vi "Test_NetworkStream Handshake.vi"() -> ()   [LabVIEW 2013]
uses:
  <vilib>/LabVIEW Open Source Project/OpenURI/utilities/Extract URI Components.vi
  <vilib>/Utility/error.llb/Trim Whitespace.vi
  <vilib>/LabVIEW Open Source Project/Unicity/RandomStringGenerator/RandomStringGenerator.lvclass
  <vilib>/LabVIEW Open Source Project/OpenURI/openURI.lvlib
panel:
  out "State verfied":bool
  out "Echo":string
  out "Echo verfied":bool
  out "Auth Ack/Nack":string
  out "Challenge verified":bool
  out "error out 2":errorcluster
  out "error out":errorcluster
  out "Client Reader":string
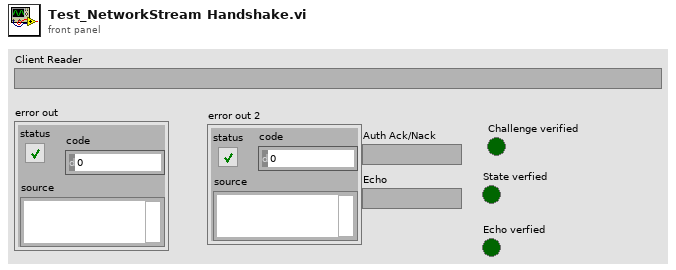
[diagram p1: front panel]
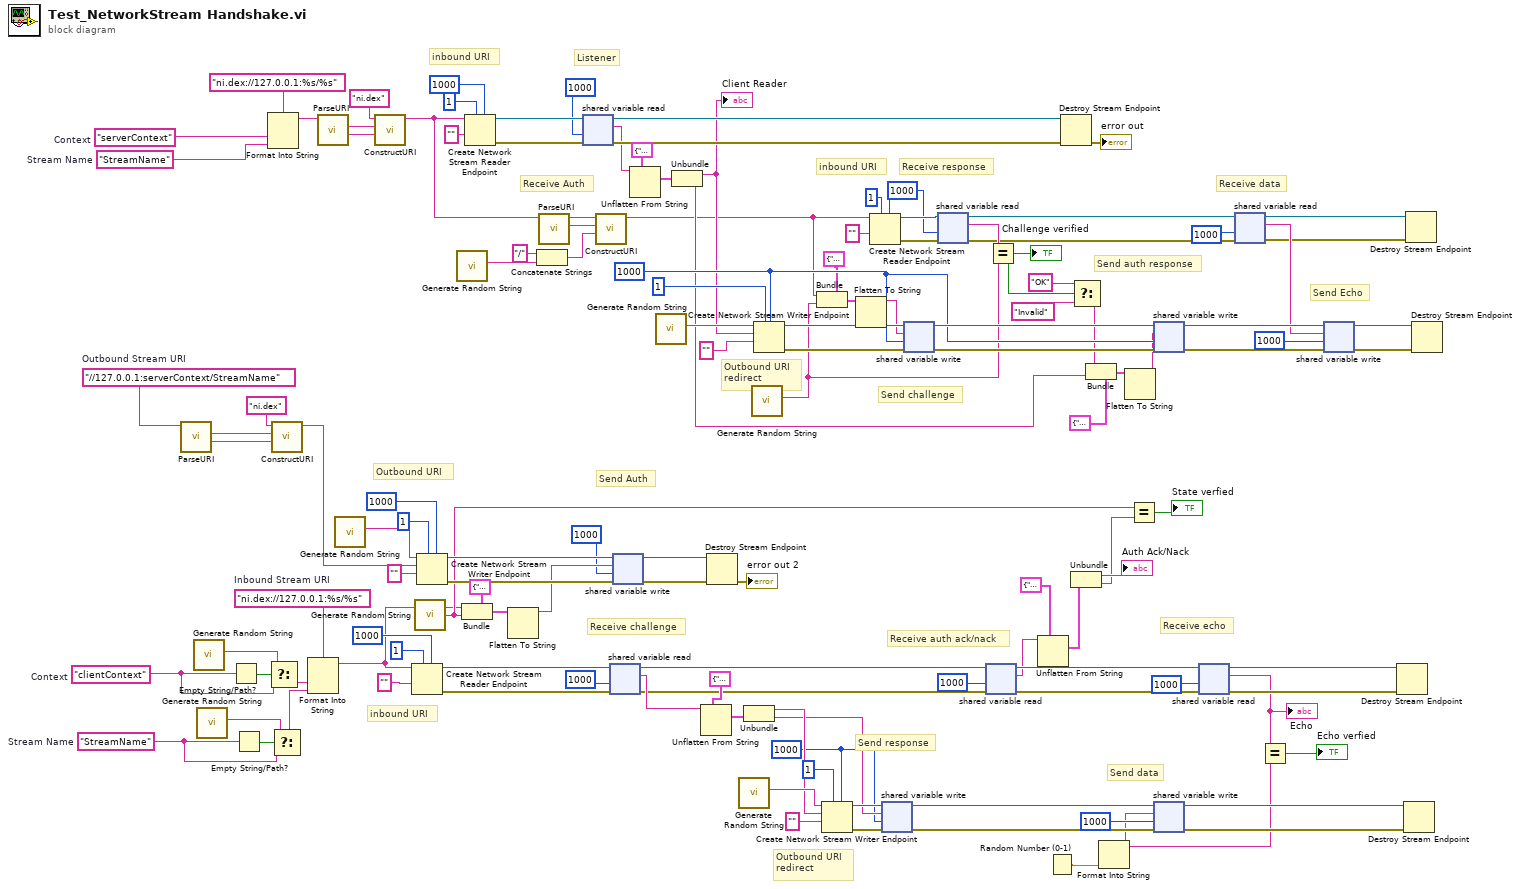
[diagram p0: block diagram]
diagram:
  w18 = "ni.dex://127.0.0.1:%s/%s"  # Inbound Stream URI
  w14 = "StreamName"  # Stream Name
  w9 = "clientContext"  # Context
  w20 = "StreamName"  # Stream Name
  w21 = "serverContext"  # Context
  w19 = "//127.0.0.1:serverContext/StreamName"  # Outbound Stream URI
  w89 = 1000 ("timeout in ms (-1)")
  w91 = 1000 ("timeout in ms (-1)")
  w83 = 1000 ("timeout in ms (-1)")
  # "Outbound URI\nredirect"
  # "Outbound URI\nredirect"
  # "Outbound URI"
  # "inbound URI"
  # "inbound URI"
  # "inbound URI"
  # "Send Echo"
  # "Receive data"
  # "Receive echo"
  # "Send data"
  # "Receive auth ack/nack"
  # "Send auth response"
  # "Receive response"
  # "Send response"
  # "Receive challenge"
  # "Send challenge"
  # "Receive Auth"
  # "Send Auth"
  # "Listener"
  n1 = call <vilib>:"ParseURI.vi"("URI"=w19) -> ("path"=w28:string, "authority"=w29:string)  [unwired: 5 in, 4 out]
  n2 = call <vilib>:"Generate Random String.vi"() -> ("Random String"=w12:string)  [unwired: 11 in]
  n3 = call <vilib>:"Generate Random String.vi"() -> ("Random String"=w15:string)  [unwired: 11 in]
  n4 = Empty String/Path?(string/path=w9) -> (empty?=w11:bool)
  n5 = Empty String/Path?(string/path=w14) -> (empty?=w16:bool)
  n6 = Format Into String(format string="ni.dex://127.0.0.1:%s/%s", w21, w20) -> (resulting string=w23:string)  [unwired: 2 in, 1 out]
  n7 = Select(t=w12, s=w11, f=w9) -> (s? t:f=w10:string)
  n8 = call <vilib>:"ConstructURI.vi"("path component"=w28, "authority"=w29, "scheme"="ni.dex" ("reader name")) -> ("URI"=w26:string)  [unwired: 7 in, 1 out]
  n9 = Select(t=w15, s=w16, f=w14) -> (s? t:f=w13:string)
  n10 = Format Into String(format string=w18, w10, w13) -> (resulting string=w17:string)  [unwired: 2 in, 1 out]
  n11 = call <vilib>:"ParseURI.vi"("URI"=w23) -> ("path"=w24:string, "authority"=w4:string)  [unwired: 5 in, 4 out]
  n12 = call <vilib>:"Generate Random String.vi"() -> ("Random String"=w114:string)  [unwired: 11 in]
  n13 = call <vilib>:"ConstructURI.vi"("path component"=w24, "authority"=w4, "scheme"="ni.dex" ("reader name")) -> ("URI"=w1:string)  [unwired: 7 in, 1 out]
  n14 = Create Network Stream Reader Endpoint(5:1000 ("timeout in ms (-1)"), 7:1 ("reader buffer size"), 9:"", 11:w17) -> (0:w46:errorcluster, 3:w117:refnum<k21>)  [unwired: 3 in]
  n15 = call <vilib>:"Generate Random String.vi"() -> ("Random String"=w30:string)  [unwired: 11 in]
  n16 = Create Network Stream Writer Endpoint(5:1000 ("timeout in ms (-1)"), 7:1 ("reader buffer size"), 9:"", 10:w26, 11:w114) -> (0:w124:errorcluster, 3:w126:refnum<k21>)  [unwired: 2 in]
  n17 = call <vilib>:"Generate Random String.vi"() -> ("Random String"=w8:string)  [unwired: 11 in]
  n18 = Bundle(cluster=cluster{"uri":string, "header":string} {"uri"="", "header"=""}, "uri"=w17, "header"=w30) -> (w45:cluster{"uri":string, "header":string})
  n19 = Create Network Stream Reader Endpoint(5:1000 ("timeout in ms (-1)"), 7:1 ("reader buffer size"), 9:"", 11:w1) -> (0:w131:errorcluster, 3:w132:refnum<k21>)  [unwired: 3 in]
  n20 = Flatten To String(anything=w45) -> (data string=w109:string)  [unwired: 3 in, 2 out]
  n21 = Concatenate Strings("/" ("string"), w8) -> (w3:string)
  n22 = call <vilib>:"ParseURI.vi"("URI"=w1) -> ("authority"=w5:string, "scheme"=w6:string)  [unwired: 5 in, 4 out]
  n23 = shared-variable-read(w132, w131, 1000 ("timeout in ms (-1)")) -> (w129:refnum<k21>, w128:errorcluster, w110:string)  [unwired: 1 out]
  n24 = call <vilib>:"ConstructURI.vi"("path component"=w3, "authority"=w5, "scheme"=w6) -> ("URI"=w2:string)  [unwired: 7 in, 1 out]
  n25 = shared-variable-read(w117, w46, 1000 ("timeout in ms (-1)")) -> (w82:refnum<k21>, w62:errorcluster, w98:string)  [unwired: 1 out]
  n26 = shared-variable-write(w126, w124, w109, 1000 ("timeout in ms (-1)")) -> (w106:refnum<k21>, w105:errorcluster)  [unwired: 1 out]
  n27 = Unflatten From String(type=cluster{"uri":string, "header":string} {"uri"="", "header"=""} ("cluster"), binary string=w110) -> (value=w43:cluster{"uri":string, "header":string})  [unwired: 3 in, 2 out]
  n28 = call <vilib>:"Generate Random String.vi"() -> ("Random String"=w115:string)  [unwired: 11 in]
  n29 = Unbundle(w43) -> ("uri"=w42:string, "header"=w37:string)
  "Client Reader" <- w42
  n30 = Unflatten From String(type=cluster{"redirect":string, "challenge":string} {"redirect"="", "challenge"=""} ("cluster"), binary string=w98) -> (value=w97:cluster{"redirect":string, "challenge":string})  [unwired: 3 in, 2 out]
  n31 = Destroy Stream Endpoint(8:w105, 11:w106) -> (0:→"error out 2":errorcluster)
  n32 = call <vilib>:"Generate Random String.vi"() -> ("Random String"=w104:string)  [unwired: 11 in]
  n33 = Unbundle(w97) -> ("redirect"=w96:string, "challenge"=w94:string)
  n34 = call <vilib>:"Generate Random String.vi"() -> ("Random String"=w51:string)  [unwired: 11 in]
  n35 = Create Network Stream Writer Endpoint(5:w83, 7:1 ("reader buffer size"), 9:"", 10:w42, 11:w115) -> (0:w113:errorcluster, 3:w118:refnum<k21>)  [unwired: 2 in]
  n36 = Bundle(cluster=cluster{"redirect":string, "challenge":string} {"redirect"="", "challenge"=""}, "redirect"=w2, "challenge"=w51) -> (w101:cluster{"redirect":string, "challenge":string})
  n37 = Create Network Stream Writer Endpoint(5:w89, 7:1 ("reader buffer size"), 9:"", 10:w96, 11:w104) -> (0:w57:errorcluster, 3:w95:refnum<k21>)  [unwired: 2 in]
  n38 = Flatten To String(anything=w101) -> (data string=w100:string)  [unwired: 3 in, 2 out]
  n39 = Create Network Stream Reader Endpoint(5:w91, 7:1 ("reader buffer size"), 9:"", 11:w2) -> (0:w92:errorcluster, 3:w93:refnum<k21>)  [unwired: 3 in]
  n40 = shared-variable-write(w95, w57, w94, w89) -> (w78:refnum<k21>, w58:errorcluster)  [unwired: 1 out]
  n41 = shared-variable-write(w118, w113, w100, w83) -> (w88:refnum<k21>, w87:errorcluster)  [unwired: 1 out]
  n42 = shared-variable-read(w93, w92, w91) -> (w73:refnum<k21>, w71:errorcluster, w90:string)  [unwired: 1 out]
  n43 = shared-variable-read(w82, w62, 1000 ("timeout in ms (-1)")) -> (w76:refnum<k21>, w61:errorcluster, w36:string)  [unwired: 1 out]
  n44 = Equal?(x=w90, y=w51) -> (x = y?=w86:bool)
  "Challenge verified" <- w86
  n45 = Unflatten From String(type=cluster{"response":string, "header":string} {"response"="", "header"=""} ("cluster"), binary string=w36) -> (value=w34:cluster{"response":string, "header":string})  [unwired: 3 in, 2 out]
  n46 = Random Number (0-1)() -> (number: 0 to 1=w80:dbl)
  n47 = Destroy Stream Endpoint(8:w128, 11:w129) -> (0:→"error out":errorcluster)
  n48 = Unbundle(w34) -> ("response"=→"Auth Ack/Nack":string, "header"=w32:string)
  n49 = Select(t="OK", s=w86, f="Invalid") -> (s? t:f=w39:string)
  n50 = Bundle(cluster=cluster{"response":string, "header":string} {"response"="", "header"=""}, "response"=w39, "header"=w37) -> (w40:cluster{"response":string, "header":string})
  n51 = Format Into String(w80) -> (resulting string=w55:string)  [unwired: 3 in, 1 out]
  n52 = Flatten To String(anything=w40) -> (data string=w38:string)  [unwired: 3 in, 2 out]
  n53 = Equal?(x=w30, y=w32) -> (x = y?=→"State verfied":bool)
  n54 = shared-variable-write(w88, w87, w38, w83) -> (w68:refnum<k21>, w70:errorcluster)  [unwired: 1 out]
  n55 = shared-variable-write(w78, w58, w55, 1000 ("timeout in ms (-1)")) -> (w77:refnum<k21>, w59:errorcluster)  [unwired: 1 out]
  n56 = shared-variable-read(w76, w61, 1000 ("timeout in ms (-1)")) -> (w75:refnum<k21>, w60:errorcluster, w56:string)  [unwired: 1 out]
  "Echo" <- w56
  n57 = shared-variable-read(w73, w71, 1000 ("timeout in ms (-1)")) -> (w64:refnum<k21>, w63:errorcluster, w66:string)  [unwired: 1 out]
  n58 = Equal?(x=w56, y=w55) -> (x = y?=→"Echo verfied":bool)
  n59 = shared-variable-write(w68, w70, w66, 1000 ("timeout in ms (-1)")) -> (w67:refnum<k21>, w69:errorcluster)  [unwired: 1 out]
  n60 = Destroy Stream Endpoint(8:w60, 11:w75) -> ()  [unwired: 1 out]
  n61 = Destroy Stream Endpoint(8:w59, 11:w77) -> ()  [unwired: 1 out]
  n62 = Destroy Stream Endpoint(8:w63, 11:w64) -> ()  [unwired: 1 out]
  n63 = Destroy Stream Endpoint(8:w69, 11:w67) -> ()  [unwired: 1 out]
